vi "ExSubCreateDataStrip.vi"(0 "Camera Handle":u32, 1 "error in (no error)":errorcluster) -> (2 "Camera Handle":u32, 3 "Data/Image Handle":u32, 4 "error out":errorcluster)   [LabVIEW 2010]
panel:
  # "ExSubCreateDataStrip:\nThis Sub-VI creates a Data handle for data collection"
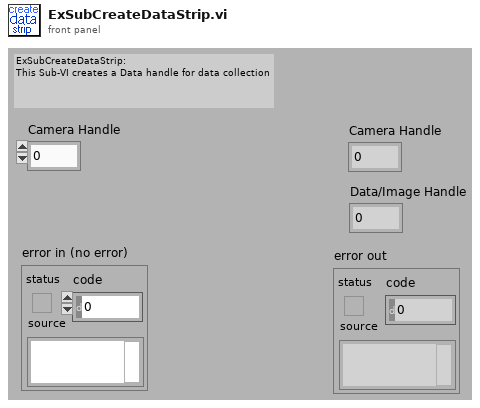
[diagram p1: front panel]
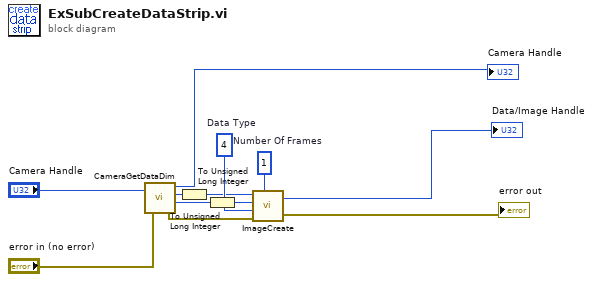
[diagram p0: block diagram]
diagram:
  w6 = u32 4  # Data Type
  w7 = u32 1  # Number Of Frames
  n1 = call <userlib>:"CameraGetDataDim.vi"("Camera Handle"="Camera Handle", "error in"="error in (no error)") -> ("Camera Handle"=→"Camera Handle":u32, "Xdim"=w10:u32, "Ydim"=w11:u32, "error out"=w12:errorcluster)
  n2 = To Unsigned Long Integer(number=w10) -> (unsigned 32bit integer=w5:u32)
  n3 = To Unsigned Long Integer(number=w11) -> (unsigned 32bit integer=w4:u32)
  n4 = call <userlib>:"ImageCreate.vi"("X dimension"=w5, "Y dimension"=w4, "Data Type"=w6, "error in"=w12, "Number Of Frames"=w7) -> ("Image Handle"=→"Data/Image Handle":u32, "error out"=→"error out":errorcluster)
